vi "saveData2CSV.vi"(7 "append header file":bool, 8 "append to file":bool, 9 "Data in":string[][](array[string]), 10 "Header file":string[](array[string]), 11 "file path in":path) -> (3 "file path out":path)   [LabVIEW 2011]
uses:
  <vilib>/Utility/file.llb/Write To Spreadsheet File (string).vi
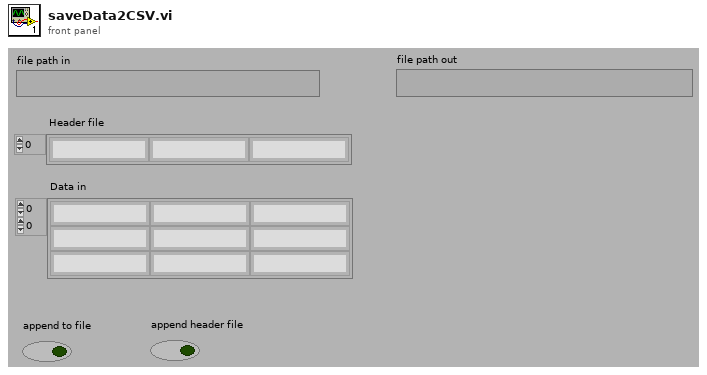
[diagram p1: front panel]
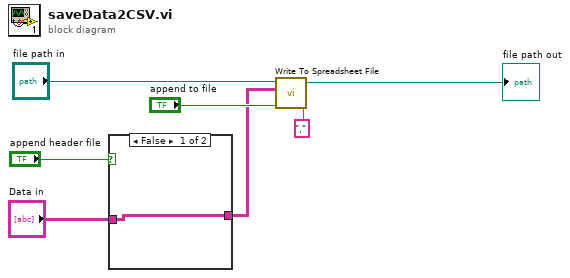
[diagram p0: block diagram]
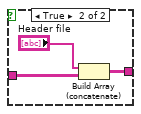
[diagram p2: hidden frame]
diagram:
  n1 = case shown="False" "append header file" {
    tunnel: "Data in" -> [w8 w11]
    tunnel: [w8 w9] -> w2
    frame False {
    }
    frame True {
      n2 = Build Array (concatenate)("Header file", w11) -> (w9:string[][])
    }
  }
  n3 = call-poly <vilib>:"Write To Spreadsheet File.vi"("delimiter (\\t)"="," ("delimiter (\\t)"), "append to file? (new file:F)"="append to file", "2D data"=w2, "file path (dialog if empty)"="file path in") -> ("new file path (Not A Path if cancelled)"=→"file path out":path)  [unwired: 4 in]
